vi "Tecan Mngr.vi"(0 "Address":u8, 1 "Mngr Action":T7, 5 "Cmd":string, 7 "Pump Data":T4={"Syringe Pos"=0, "Rate"=0.0, "Volume"=0.0, "Valve"=enum."Bottle 1", "Action"=enum."Withdraw", "Move Type"=enum."Rel", "Init"=TRUE, "Empty Syr."=TRUE, "Full Fill"=TRUE, "Units"=enum."ul/s"} {"Syringe Pos" scale=0.0..100.0}, 9 "Pump Config":T1={"Syringe size"=0, "Syringe address"=0, "# of ports"=0, "Init String"="", "Full Stroke (cnts)"=0, "Model"=enum."XC", "TW Position"=0.0, "Load Position"=0.0, "Bottom Position"=0.0, "Station ID"="", "Default Protocol"=path "", "Dry Time(s)"=0.0, "Python Version"="", "NFC SN Array"=["21121521200223", "21121521200186", "21121521200213", "52541737200062"], "Timing"={"Checking pres and leak"=0.0, "Priming input lines"=0.0, "Rinsing syringe"=0.0, "Filling well X w/ X"=0.0, "Drain well X"=0.0, "Clearing wells and lines"=0.0, "Draining wells"=0.0, "Rinsing all wells"=0.0, "Testing for leaks/clogs"=0.0, "Rinsing wells"=0.0}, "Pressure Specs"={"Pressure max"=0.0, "Pressure min"=0.0, "Decay delta"=0.0, "Pressure time"=0.0, "Conf. R"=0.0, "LeakRateMax"=0.0}}, 11 "error in (no error)":errorcluster, 12 "Valve":enum16{"Input", "Output"}(ring)) -> (6 "Raw Response":string, 8 "Output Value":dbl caption="Current Position(half steps)", 10 "Error Code":string, 13 "Move Successful":bool, 14 "Connected":bool, 15 "error out":errorcluster)   [LabVIEW 2020]
uses:
  Tricon Mngr.ctl
  Tecan/Pump Control.ctl
  Main/Pump Port.ctl
  Tecan/Velocity Units.ctl
  Tecan/Pump Config.ctl
  Main/Timing Specs.ctl
  Main/Vacuum Specs.ctl
  Lib/Serial/Find Device Protocols.ctl
  Tecan/Pump Direction.ctl
  Hardware Globals.vi
  Lib/Utilities.lvlib
panel:
  # "Tecan Pump"
  # "Pressure"
  # "General"
  # "Timing"
  # "Protocol"
  # "Zaber"
  # "NFC Reader 1"
  # "NFC  Reader 2"
  # "NFC Reader 3"
  # "NFC Reader 4"
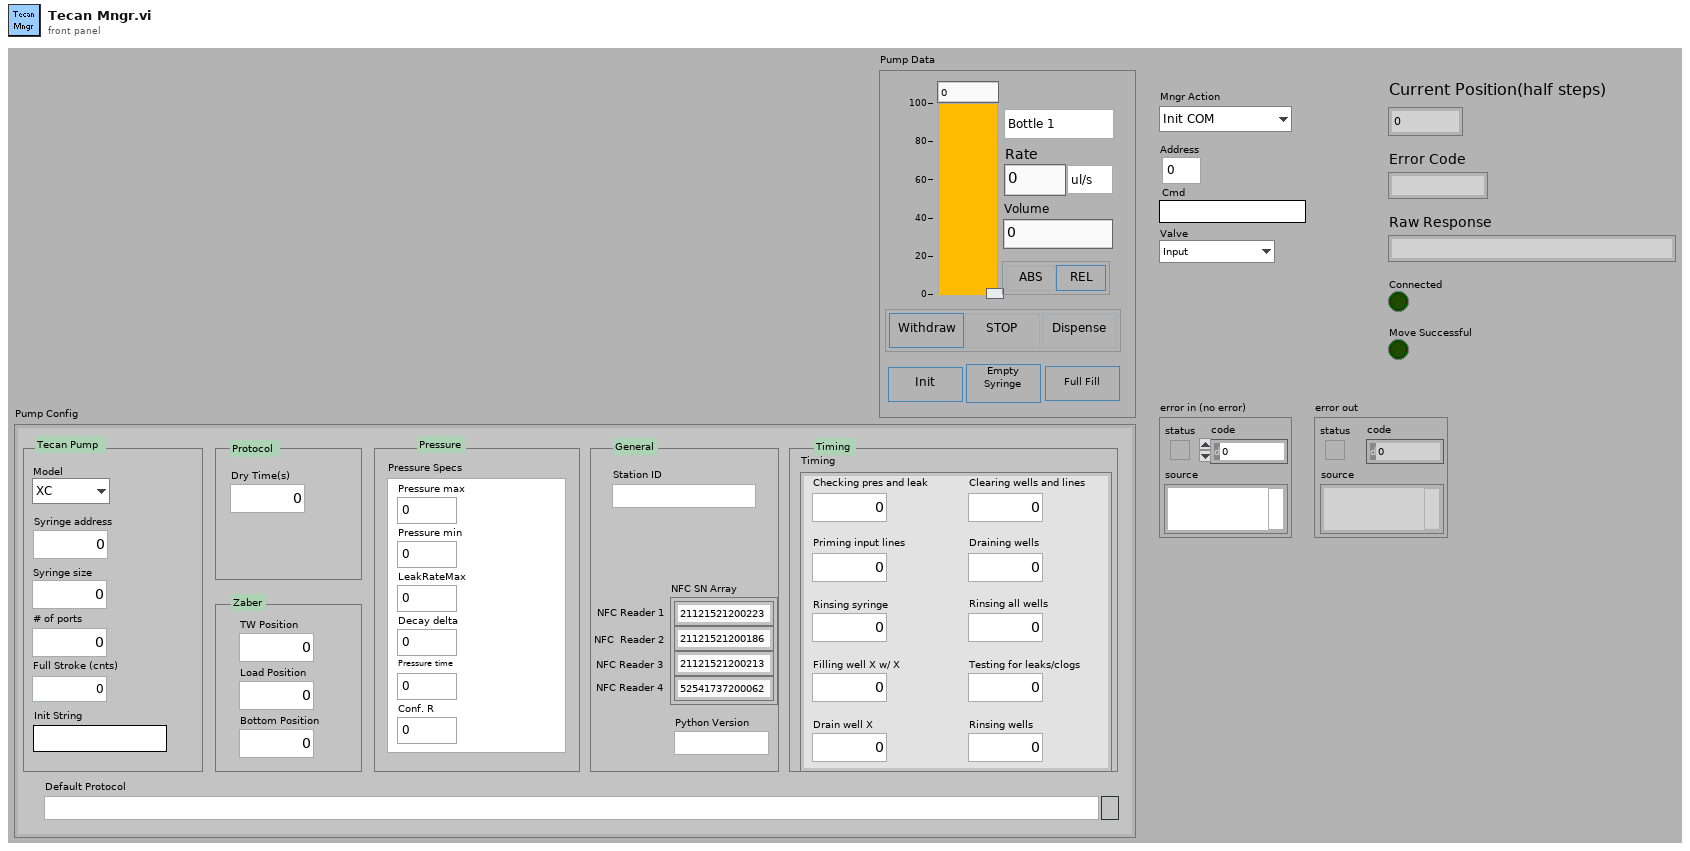
[diagram p1: front panel]
types:
  T1 = typedef "Pump Config.ctl" = cluster{"Syringe size":u32, "Syringe address":u32, "# of ports":u32, "Init String":string, "Full Stroke (cnts)":i32, "Model":enum16{"XC", "Centris"}, "TW Position":dbl, "Load Position":dbl, "Bottom Position":dbl, "Station ID":string, "Default Protocol":path, "Dry Time(s)":dbl, "Python Version":string, "NFC SN Array":string[], "Timing":T2, "Pressure Specs":T3}
  T2 = typedef "Timing Specs.ctl" = cluster{"Checking pres and leak":dbl, "Priming input lines":dbl, "Rinsing syringe":dbl, "Filling well X w/ X":dbl, "Drain well X":dbl, "Clearing wells and lines":dbl, "Draining wells":dbl, "Rinsing all wells":dbl, "Testing for leaks/clogs":dbl, "Rinsing wells":dbl}
  T3 = typedef "Vacuum Specs.ctl" = cluster{"Pressure max":dbl, "Pressure min":dbl, "Decay delta":dbl, "Pressure time":dbl, "Conf. R":dbl, "LeakRateMax":dbl}
  T4 = typedef "Pump Control.ctl" = cluster{"Syringe Pos":u32, "Rate":dbl, "Volume":dbl, "Valve":T5, "Action":enum32{"Withdraw", "Dispense", "Stop"}, "Move Type":enum32{"Abs", "Rel"}, "Init":bool, "Empty Syr.":bool, "Full Fill":bool, "Units":T6}
  T5 = typedef "Pump Port.ctl" = enum16{"Bottle 1", "Bottle 2", "Bottle 3", "Bottle 4", "Waste", "Well 1", "Well 2", "Well 3", "Well 4", "Bottle X", "Well X"}
  T6 = typedef "Velocity Units.ctl" = enum16{"ul/s", "ul/min"}
  T7 = typedef "Tricon Mngr.ctl" = enum16{"Init COM", "Set Config", "Init Pump", "Home", "Cmd", "Start Pump", "Set Valve", "Dispense", "Withdraw", "Status", "Close"}
  T8 = typedef "Find Device Protocols.ctl" = enum16{"Init", "RS232(no baud)", "RS232", "RS485", "USB", "GPIB", "Ethernet"}
  T9 = enum16{"Init", "Reset", "Read", "Update", "Close"}
  T10 = typedef "Pump Direction.ctl" = enum16{"Dispense", "Withdraw", "Stop"}
  T11 = cluster{"negative limit switch":bool, "positive limit switch":bool, "home switch":bool, "position marker":bool, "device enable":bool, "quick stop":bool, "general purpose J":bool, "general purpose I":bool, "general purpose H":bool, "general purpose G":bool, "general purpose F":bool, "general purpose E":bool, "general purpose D":bool, "general purpose C":bool, "general purpose B":bool, "general purpose A":bool}
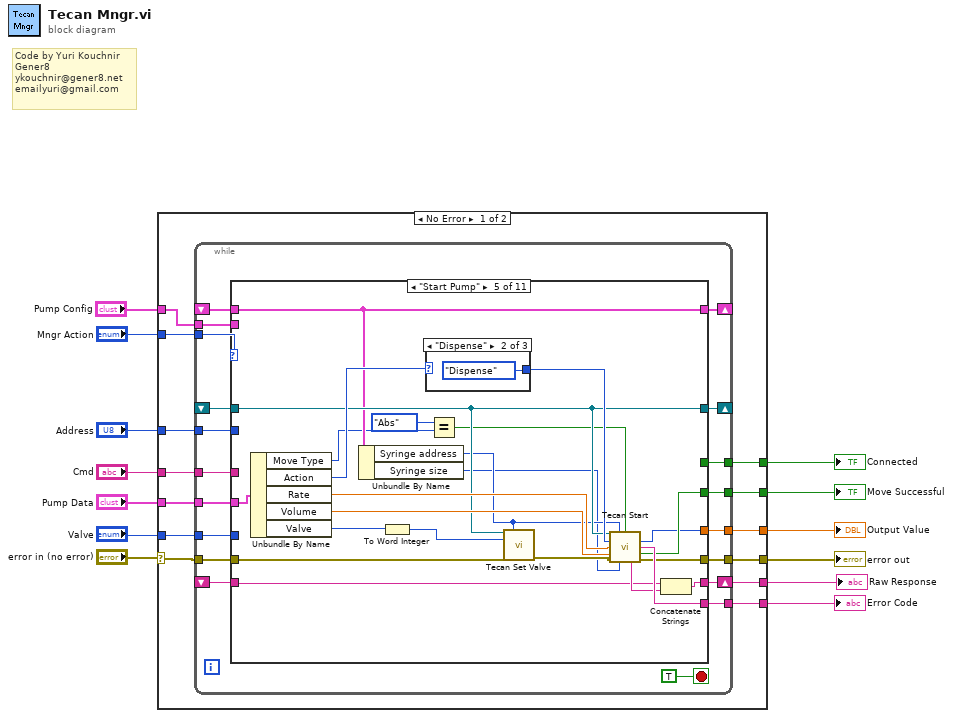
[diagram p0: block diagram]
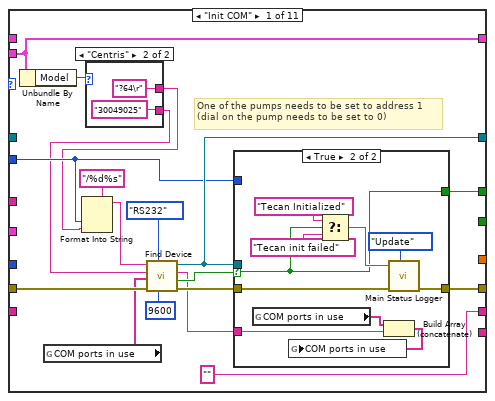
[diagram p2: hidden frame]
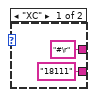
[diagram p3: hidden frame]
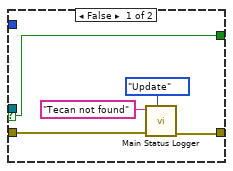
[diagram p4: hidden frame]
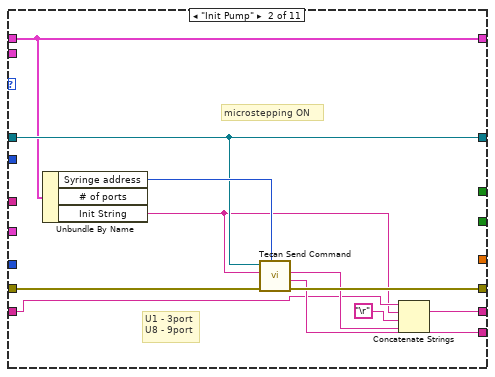
[diagram p5: hidden frame]
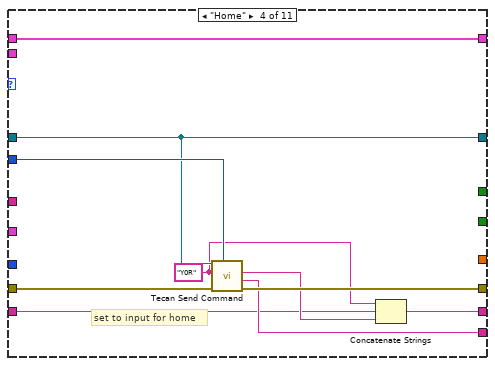
[diagram p7: hidden frame]
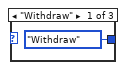
[diagram p8: hidden frame]
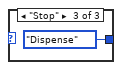
[diagram p9: hidden frame]
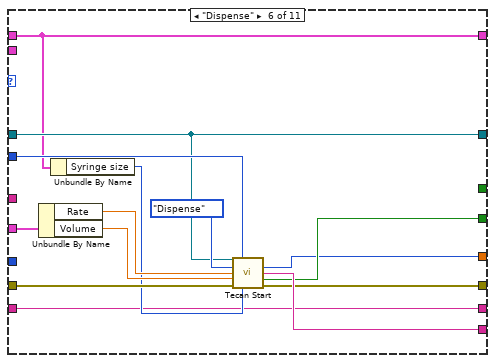
[diagram p10: hidden frame]
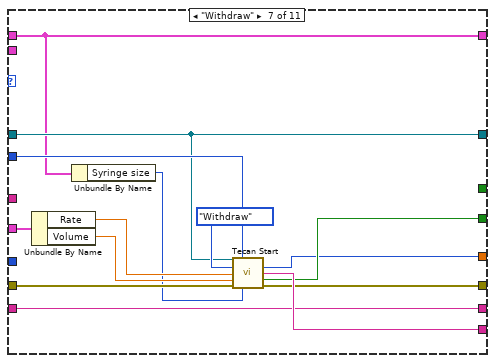
[diagram p11: hidden frame]
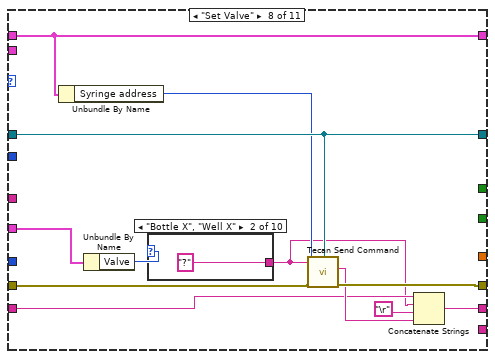
[diagram p12: hidden frame]
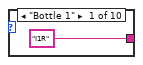
[diagram p13: hidden frame]
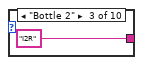
[diagram p14: hidden frame]
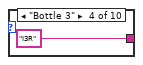
[diagram p15: hidden frame]
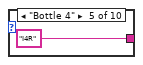
[diagram p16: hidden frame]
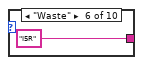
[diagram p17: hidden frame]
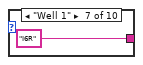
[diagram p18: hidden frame]
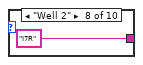
[diagram p19: hidden frame]
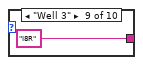
[diagram p20: hidden frame]
diagram:
  # "Code by Yuri Kouchnir\nGener8\nykouchnir@gener8.net\nemailyuri@gmail.com"
  n1 = case shown="No Error" "error in (no error)" {
    selector: "error in (no error)" -> [w26 w218]
    tunnel: [w25 w218] -> w12
    tunnel: "Mngr Action" -> [w24 _]
    tunnel: [w23 _] -> w10
    tunnel: "Address" -> [w22 _]
    tunnel: [w21 _] -> w9
    tunnel: [w20 _] -> w8
    tunnel: [w19 _] -> w7
    tunnel: "Cmd" -> [w18 _]
    tunnel: [w17 _] -> w5
    tunnel: "Valve" -> [w16 _]
    tunnel: "Pump Data" -> [w15 _]
    tunnel: "Pump Config" -> [w14 _]
    frame No Error {
      n2 = while {
        tunnel: w26 -> [w43]
        tunnel: [w42] -> w25
        tunnel: w24 -> [w44]
        tunnel: [w41] -> w23
        shift-right: [w40] -> _
        shift-left: _ -> [w39]
        tunnel: w22 -> [w38]
        tunnel: [w37] -> w21
        tunnel: [w36] -> w20
        tunnel: [w35] -> w19
        tunnel: w18 -> [w34]
        tunnel: w16 -> [w32]
        tunnel: w15 -> [w31]
        shift-right: [w30] -> _
        shift-left: _ -> [w28]
        tunnel: w14 -> [w29]
        shift-right: [w33] -> w17
        shift-left: _ -> [w27]
        stop <- TRUE stop-if-true
        n3 = case shown="\"Start Pump\"" w44 {
          tunnel: w43 -> [w62 w89 w95 w102 w120 w147 w161 w173 w195 w206 w217]
          tunnel: [w63 w93 w95 w105 w129 w143 w157 w172 w194 w205 w216] -> w42
          tunnel: [w59 _ _ _ _ _ _ _ _ _ _] -> w41
          tunnel: [w58 w90 w96 w106 w119 w142 w156 w171 w193 w204 w213] -> w40
          tunnel: w39 -> [_ w90 w96 w106 w119 w142 w156 w171 w193 w204 w213]
          tunnel: w38 -> [w50 _ _ w107 _ w146 w160 _ w192 _ _]
          tunnel: [_ w92 _ w104 w130 w144 w158 _ w189 _ _] -> w37
          tunnel: [_ _ _ _ w128 w141 w155 _ _ _ _] -> w36
          tunnel: [_ _ _ _ w127 w140 w154 _ w187 w203 _] -> w35
          tunnel: w34 -> [_ _ _ _ _ _ _ _ _ w197 _]
          tunnel: ["" ("ID Response") w87 w94 w99 w115 w134 w148 w165 w186 w201 w207] -> w33
          tunnel: w32 -> [_ _ _ _ _ _ _ _ _ _ _]
          tunnel: w31 -> [_ _ _ _ w126 w139 w153 w170 _ _ _]
          tunnel: [w49 w83 w97 w103 w118 w136 w150 w169 w188 w200 w214] -> w30
          tunnel: w29 -> [w49 _ w97 _ _ _ _ _ _ _ _]
          tunnel: w28 -> [_ w83 _ w103 w118 w136 w150 w169 w188 w200 w214]
          tunnel: w27 -> [_ w86 w94 w100 w113 w134 w148 w164 w184 w198 w207]
          frame "Init COM" {
            # "One of the pumps needs to be set to address 1\n(dial on the pump needs to be set to 0)"
            n4 = Unbundle By Name(w49) -> ("Model"=w48:enum16{"XC", "Centris"})
            n5 = global read "Hardware Globals.vi" "COM ports in use"() -> (w52:string[])
            n6 = case shown="\"Centris\"" w48 {
              tunnel: ["#\r" ("ID Response") "?64\r" ("ID Response")] -> w46
              tunnel: ["18111" ("ID Response") "30049025" ("ID Response")] -> w47
              frame "XC" {
              }
              frame "Centris" {
              }
            }
            n7 = Format Into String(format string="/%d%s" ("ID String"), w50, w46) -> (resulting string=w54:string)  [unwired: 2 in, 1 out]
            n8 = call "Find Device.vi"("Baud Rate"=u32 9600, "Device Type"=Find_Device_Protocols."RS232", "error in (no error)"=w62, "Ports in Use"=w52, "ID Response"=w47, "ID String"=w54) -> ("error out"=w61:errorcluster, "Device Found"=w60:bool, "device ID"=w53:string, "VISA resource name out"=w58:refnum<visa-resource-name>)  [unwired: 1 in, 1 out]
            n9 = case shown="True" w60 {
              selector: w60 -> [w72 w73]
              tunnel: [w69 w78] -> w63
              tunnel: w61 -> [w70 w74]
              tunnel: [w72 w73] -> w59
              tunnel: w58 -> [_ _]
              tunnel: w53 -> [_ w75]
              tunnel: w50 -> [_ _]
              frame False {
                n10 = call "Main Status Logger.vi"("Action"=T9."Update", "error in"=w70, "Input String"="Tecan not found") -> ("error out"=w69:errorcluster)  [unwired: 7 in, 1 out]
              }
              frame True {
                n11 = global read "Hardware Globals.vi" "COM ports in use"() -> (w77:string[])
                n12 = Select(t="Tecan Initialized" ("ID Response"), s=w73, f="Tecan init failed" ("ID Response")) -> (s? t:f=w79:string)
                n13 = Build Array (concatenate)(w77, w75) -> (w76:string[])
                n14 = global write "Hardware Globals.vi" "COM ports in use"(w76) -> ()
                n15 = call "Main Status Logger.vi"("Action"=T9."Update", "error in"=w74, "Input String"=w79) -> ("error out"=w78:errorcluster)  [unwired: 7 in, 1 out]
              }
            }
          }
          frame "Init Pump" {
            # "U1 - 3port\nU8 - 9port"
            # "microstepping ON"
            n16 = Unbundle By Name(w83) -> ("Syringe address"=w91:u32, "Init String"=w84:string)  [unwired: 1 out]
            n17 = call "Tecan Send Command.vi"("Address"=w91, "error in (no error)"=w89, "Command"=w84, "VISA resource name in"=w90) -> ("error out"=w93:errorcluster, "Status Code"=w92:string, "Raw Response"=w88:string)  [unwired: 3 in, 2 out]
            n18 = Concatenate Strings(w86, w84, "\r", w88) -> (w87:string)
          }
          frame "Set Config" {
          }
          frame "Home" {
            w98 = "Y0R" ("Command")
            # "set to input for home"
            n19 = call "Tecan Send Command.vi"("Address"=w107, "error in (no error)"=w102, "Command"=w98, "VISA resource name in"=w106) -> ("error out"=w105:errorcluster, "Status Code"=w104:string, "Raw Response"=w101:string)  [unwired: 3 in, 2 out]
            n20 = Concatenate Strings(w98, w100, w101) -> (w99:string)
          }
          frame "Start Pump" {
            n21 = Unbundle By Name(w126) -> ("Move Type"=w112:enum32{"Abs", "Rel"}, "Action"=w121:enum32{"Withdraw", "Dispense", "Stop"}, "Rate"=w124:dbl, "Volume"=w123:dbl, "Valve"=w109:T5)
            n22 = Unbundle By Name(w118) -> ("Syringe address"=w117:u32, "Syringe size"=w116:u32)
            n23 = To Word Integer(number=w109) -> (16bit integer=w108:i16)
            n24 = case shown="\"Dispense\"" w121 {
              tunnel: [Pump_Direction."Withdraw" ("Direction") Pump_Direction."Dispense" ("Direction") Pump_Direction."Dispense" ("Direction")] -> w125
              frame "Withdraw" {
              }
              frame "Dispense" {
              }
              frame "Stop" {
              }
            }
            n25 = Equal?(x=enum32{"Abs", "Rel"}."Abs", y=w112) -> (x = y?=w110:bool)
            n26 = call "Tecan Set Valve.vi"("VISA resource name"=w119, "Pump Address"=w117, "Valve"=w108, "error IO"=w120) -> ("error out"=w122:errorcluster)  [unwired: 7 in, 4 out]
            n27 = call "Tecan Start.vi"("VISA resource name"=w119, "Pump Address"=w117, "Abs"=w110, "Direction"=w125, "Rate(uL/min)"=w124, "Volume(uL)"=w123, "error IO"=w122, "Syringe Capacity"=w116) -> ("Current Position(mL)"=w127:u32, "Error Code"=w130:string, "Move Successful"=w128:bool, "Response"=w114:string, "error out"=w129:errorcluster)  [unwired: 2 in, 1 out]
            n28 = Concatenate Strings(w113, w114) -> (w115:string)
          }
          frame "Dispense" {
            n29 = Unbundle By Name(w139) -> ("Rate"=w138:dbl, "Volume"=w137:dbl)
            n30 = Unbundle By Name(w136) -> ("Syringe size"=w135:u32)
            n31 = call "Tecan Start.vi"("VISA resource name"=w142, "Pump Address"=w146, "Direction"=Pump_Direction."Dispense", "Rate(uL/min)"=w138, "Volume(uL)"=w137, "error IO"=w147, "Syringe Capacity"=w135) -> ("Current Position(mL)"=w140:u32, "Error Code"=w144:string, "Move Successful"=w141:bool, "error out"=w143:errorcluster)  [unwired: 3 in, 2 out]
          }
          frame "Withdraw" {
            n32 = Unbundle By Name(w153) -> ("Rate"=w152:dbl, "Volume"=w151:dbl)
            n33 = Unbundle By Name(w150) -> ("Syringe size"=w149:u32)
            n34 = call "Tecan Start.vi"("VISA resource name"=w156, "Pump Address"=w160, "Direction"=Pump_Direction."Withdraw", "Rate(uL/min)"=w152, "Volume(uL)"=w151, "error IO"=w161, "Syringe Capacity"=w149) -> ("Current Position(mL)"=w154:u32, "Error Code"=w158:string, "Move Successful"=w155:bool, "error out"=w157:errorcluster)  [unwired: 3 in, 2 out]
          }
          frame "Set Valve" {
            n35 = Unbundle By Name(w169) -> ("Syringe address"=w168:u32)
            n36 = Unbundle By Name(w170) -> ("Valve"=w167:T5)
            n37 = case shown="\"Bottle X\", \"Well X\"" w167 {
              tunnel: ["I1R" ("Command") "?" ("Command") "I2R" ("Command") "I3R" ("Command") "I4R" ("Command") "I5R" ("Command") "I6R" ("Command") "I7R" ("Command") "I8R" ("Command") "I9R" ("Command")] -> w163
              frame "Bottle 1" {
              }
              frame "Bottle X", "Well X" {
              }
              frame "Bottle 2" {
              }
              frame "Bottle 3" {
              }
              frame "Bottle 4" {
              }
              frame "Waste" {
              }
              frame "Well 1" {
              }
              frame "Well 2" {
              }
              frame "Well 3" {
              }
              frame "Well 4" {
              }
            }
            n38 = call "Tecan Send Command.vi"("Address"=w168, "error in (no error)"=w173, "Command"=w163, "VISA resource name in"=w171) -> ("error out"=w172:errorcluster, "Raw Response"=w166:string)  [unwired: 3 in, 3 out]
            n39 = Concatenate Strings(w164, w163, "\r", w166) -> (w165:string)
          }
          frame "Status" {
            n40 = call "Tecan Send Command.vi"("Address"=w192, "error in (no error)"=w195, "Command"="?", "VISA resource name in"=w193) -> ("error out"=w194:errorcluster, "Status Code"=w189:string, "Raw Response"=w185:string, "Value"=w190:dbl)  [unwired: 3 in, 1 out]
            n41 = Concatenate Strings(w184, w185) -> (w186:string)
            n42 = To Unsigned Long Integer(number=w190) -> (unsigned 32bit integer=w187:u32)
          }
          frame "Cmd" {
            n43 = Unbundle By Name(w200) -> ("Syringe address"=w199:u32)
            n44 = call "Tecan Send Command.vi"("Address"=w199, "error in (no error)"=w206, "Command"=w197, "VISA resource name in"=w204) -> ("error out"=w205:errorcluster, "Raw Response"=w202:string, "Value"=w203:dbl)  [unwired: 3 in, 2 out]
            n45 = Concatenate Strings(w198, w197, "\r", w202) -> (w201:string)
          }
          frame "Close" {
            n46 = global read "Hardware Globals.vi" "COM ports in use"() -> (w211:string[])
            n47 = Type Cast(x=w213) -> (*(type *) &x=w212:string)  [unwired: 1 in]
            n48 = Search 1D Array(1D array=w211, element=w212) -> (index of element=w209:i32)  [unwired: 1 in]
            n49 = Delete From Array(array=w211, length=1, index=w209) -> (array with subset deleted=w208:string[])  [unwired: 1 out]
            n50 = call "Valco - Close.vi"("VISA resource name"=w213) -> ("error out"=w215:errorcluster)  [unwired: 10 in]
            n51 = global write "Hardware Globals.vi" "COM ports in use"(w208) -> ()
            n52 = Merge Errors(w215, w217) -> (w216:errorcluster)
          }
        }
      }
    }
    frame Error {
      (unwired) T11 {"negative limit switch"=FALSE, "positive limit switch"=FALSE, "home switch"=FALSE, "position marker"=FALSE, "device enable"=FALSE, "quick stop"=FALSE, "general purpose J"=FALSE, "general purpose I"=FALSE, "general purpose H"=FALSE, "general purpose G"=FALSE, "general purpose F"=FALSE, "general purpose E"=FALSE, "general purpose D"=FALSE, "general purpose C"=FALSE, "general purpose B"=FALSE, "general purpose A"=FALSE} ("digital inputs")
    }
  }
  "error out" <- w12
  "Connected" <- w10
  "Output Value" <- w7
  "Error Code" <- w9
  "Move Successful" <- w8
  "Raw Response" <- w5
